vi "Construct - Input.vi"(4 "extension":string, 5 "N Day Buffer":u32, 6 "file name format":string="Log %<%Y-%m-%d %H%M%S>T", 7 "Max File Size (MB)":dbl=512.0, 8 "Layout Type":refnum<class "Layout.lvclass">, 9 "Name":string, 10 "Level":T1=enum."DEBUG", 11 "log location":path) -> (0 "Error Out":errorcluster, 3 "Text File":refnum<class "Text File.lvclass">)   [LabVIEW 2019, in "TSC Event Logger.lvlib" / "Text File.lvclass"]
doc: "Construct a text file sink via direct entry with an output of the sink.\n\n<b>Code Developed By:</b>\nTechnology Service Corporation\nBloomington, IN 47403\nwww.tsc.com/atcs\n\nDeveloper:\nDaniel Coons"
uses:
  Text File.lvclass
  C:/Development/Open Source/tsc-event-logger/Log Sinks/Log Sinks.lvclass
  Log/Event Level.ctl
  Layouts/Layout.lvclass
  Layouts/SimpleLayout/SimpleLayout.lvclass
  C:/Development/Open Source/tsc-event-logger/Layouts/Layout.lvclass
  Text File.lvclass/Text File.ctl
  Log Sinks.lvclass/Log Sinks.ctl
  Log Sinks.lvclass
  TSC Event Logger.lvlib
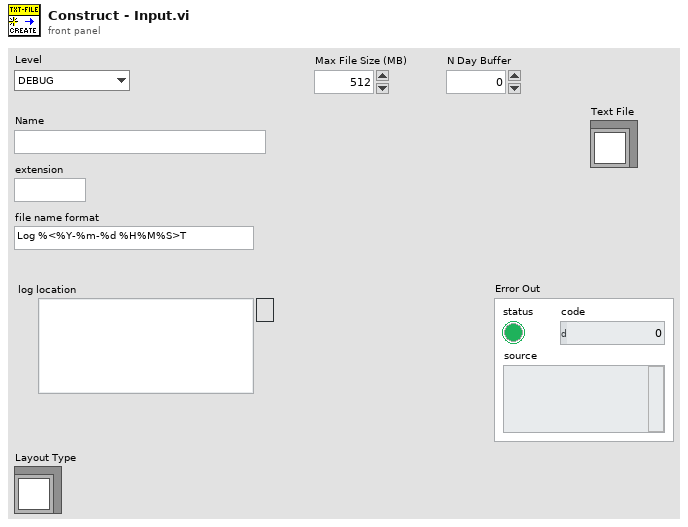
[diagram p1: front panel]
types:
  T1 = typedef "TSC Event Logger.lvlib/Event Level.ctl" = enum16{"OFF", "TRACE", "DEBUG", "INFO", "WARN", "ERROR", "FATAL"}
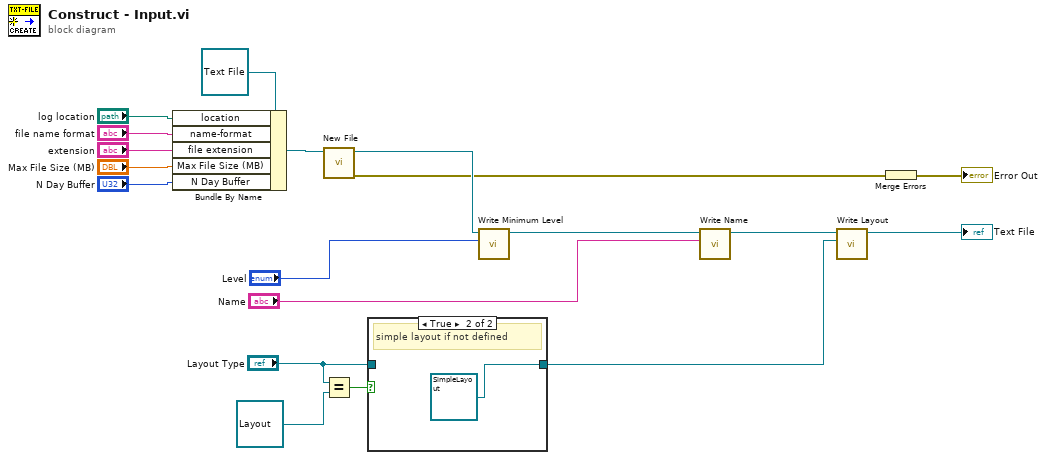
[diagram p0: block diagram]
diagram:
  n1 = Bundle By Name(cluster=refnum<class "Text File.lvclass"> refnum ("TSC Event Logger.lvlib:Text File.lvclass"), "location"="log location", "name-format"="file name format", "file extension"="extension", "Max File Size (MB)"="Max File Size (MB)", "N Day Buffer"="N Day Buffer") -> (w8:refnum<class "Text File.lvclass">)
  n2 = call "New File.vi"("Text File in"=w8) -> ("error out"=w6:errorcluster, "Text File out"=w7:refnum<class "Text File.lvclass">)  [unwired: 9 in]
  n3 = Equal?(x="Layout Type", y=refnum<class "Layout.lvclass"> refnum ("TSC Event Logger.lvlib:Layout.lvclass")) -> (x = y?=w4:bool)
  n4 = case shown="True" w4 {
    tunnel: "Layout Type" -> [w20 _]
    tunnel: [w20 refnum<class "SimpleLayout.lvclass"> refnum ("TSC Event Logger.lvlib:SimpleLayout.lvclass")] -> w2
    frame False {
    }
    frame True {
      # "simple layout if not defined"
    }
  }
  n5 = call "Write Minimum Level.vi"("Level"="Level", "Log Sinks in"=w7) -> ("Log Sinks out"=w19:refnum<class "Text File.lvclass">)  [unwired: 9 in]
  n6 = call "Write Name.vi"("Name"="Name", "Log Sinks in"=w19) -> ("Log Sinks out"=w18:refnum<class "Text File.lvclass">)  [unwired: 9 in]
  n7 = call "Write Layout.vi"("Layout"=w2, "Log Sinks in"=w18) -> ("Log Sinks out"=→"Text File":refnum<class "Text File.lvclass">)  [unwired: 9 in]
  n8 = Merge Errors(w6) -> (→"Error Out":errorcluster)
